vi "Finish.vi"   [LabVIEW 2019]
doc: "This VI is called just before exiting. It is expected to close I/O refnum, save collected data, etc."
uses:
  RefNums_Actuators.vi
  Joystick RefNum.vi
  RefNums_Sensors.vi
types:
  T1 = typedef "WPI_MotorControlDeviceRef.ctl" = cluster{"DeviceStatus":errorcluster, "Type":T2, "PWM":cluster{"PWM Channel":T3, "DeadBand":T4}, "CAN":cluster{"Device Number":u8, "SetOutput VI Ref":variant, "GetOutput VI Ref":variant, "Enable VI Ref":variant, "Disable VI Ref":variant, "Data":variant}, "Invert":bool, "DIO PWM":cluster{"PWM \"Enable\" Channel":T3, "DIOChannel":T5, "PWM Rate":dbl}}
  T2 = typedef "WPI_MotorControlType.ctl" = enum16{"PWM", "CAN", "DIO PWM"}
  T3 = typedef "FPGA_DIOPWMChannel.ctl" = enum8{"PWM 0", "PWM 1", "PWM 2", "PWM 3", "PWM 4", "PWM 5", "PWM 6", "PWM 7", "PWM 8", "PWM 9", "PWM MXP 0", "PWM MXP 1", "PWM MXP 2", "PWM MXP 3", "PWM MXP 4", "PWM MXP 5", "PWM MXP 6", "PWM MXP 7", "PWM MXP 8", "PWM MXP 9", "Invalid"}
  T4 = typedef "WPI_PWMDeadband.ctl" = cluster{"Name":string, "maxPositivePwm":i32, "minPositivePwm":i32, "centerPwm":i32, "maxNegativePwm":i32, "minNegativePwm":i32, "angularRange":u16}
  T5 = typedef "FPGA_DIOChannel.ctl" = enum8{"DIO 0", "DIO 1", "DIO 2", "DIO 3", "DIO 4", "DIO 5", "DIO 6", "DIO 7", "DIO 8", "DIO 9", "DIO MXP 0", "DIO MXP 1", "DIO MXP 2", "DIO MXP 3", "DIO MXP 4", "DIO MXP 5", "DIO MXP 6", "DIO MXP 7", "DIO MXP 8", "DIO MXP 9", "DIO MXP 10", "DIO MXP 11", "DIO MXP 12", "DIO MXP 13", "DIO MXP 14", "DIO MXP 15", "SPI Port CS1", "SPI Port CS2", "SPI Port CS3", "SPI Port MISO", "SPI Port MOSI", "Invalid"}
  T6 = typedef "WPI_JoystickDevRef.ctl" = cluster{"Device":T7}
  T7 = typedef "WPI_JoystickDeviceEnum.ctl" = enum16{"USB 0", "USB 1", "USB 2", "USB 3", "USB 4", "USB 5"}
  T8 = typedef "WPI_CompressorDevRef.ctl" = cluster{"DevStatus":errorcluster, "Pneumatics Control Module":u8}
  T9 = typedef "WPI_SolenoidDevRef.ctl" = cluster{"DevStatus":errorcluster, "Pneumatics Control Module":u8, "Forward Solenoid Channel":T10, "Reverse Solenoid Channel":T10}
  T10 = typedef "WPI_SolenoidChannel.ctl" = enum8{"Solenoid 0", "Solenoid 1", "Solenoid 2", "Solenoid 3", "Solenoid 4", "Solenoid 5", "Solenoid 6", "Solenoid 7", "Invalid"}
  T11 = typedef "WPI_AnalogChannelDevRef.ctl" = cluster{"DevStatus":errorcluster, "Analog Channel":T12}
  T12 = typedef "FPGA_AIChannel.ctl" = enum8{"AI 0", "AI 1", "AI 2", "AI 3", "AI MXP 0", "AI MXP 1", "AI MXP 2", "AI MXP 3", "Invalid"}
  T13 = typedef "WPI_ServoDeviceRef.ctl" = cluster{"DeviceStatus":errorcluster, "PWM Channel":T3, "DeadBand":T4}
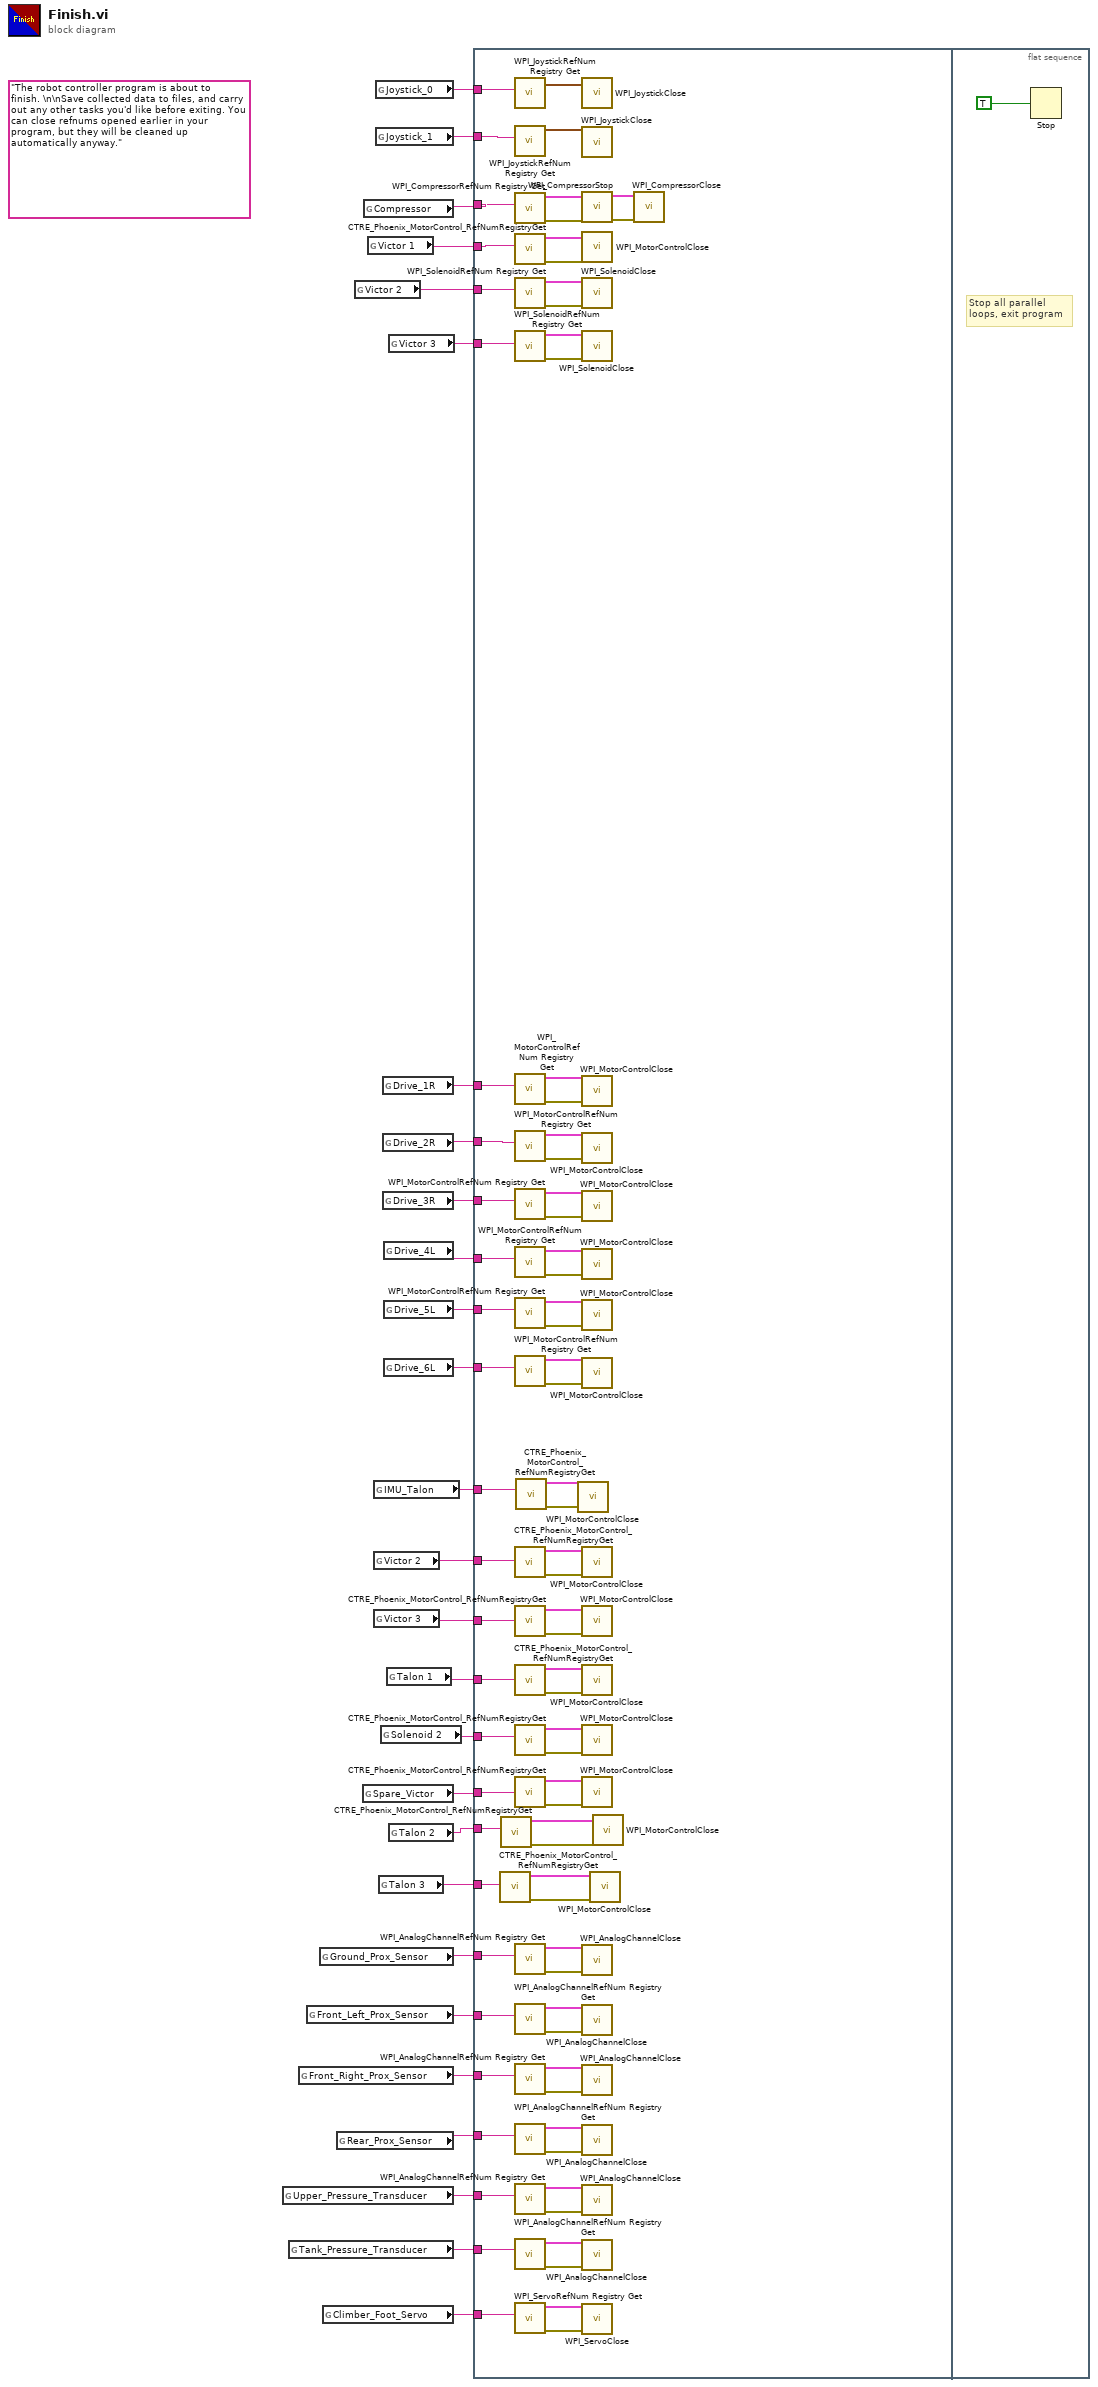
[diagram p0: block diagram]
diagram:
  (unwired) "The robot controller program is about to finish. \n\nSave collected data to files, and carry out any other tasks you'd like before exiting. You can close refnums opened earlier in your program, but they will be cleaned up automatically anyway."
  n1 = global read "RefNums_Sensors.vi" "Upper_Pressure_Transducer"() -> (w7:string)
  n2 = global read "RefNums_Sensors.vi" "Tank_Pressure_Transducer"() -> (w6:string)
  n3 = global read "RefNums_Sensors.vi" "Front_Right_Prox_Sensor"() -> (w9:string)
  n4 = global read "RefNums_Sensors.vi" "Front_Left_Prox_Sensor"() -> (w10:string)
  n5 = global read "RefNums_Sensors.vi" "Ground_Prox_Sensor"() -> (w24:string)
  n6 = global read "RefNums_Actuators.vi" "Climber_Foot_Servo"() -> (w23:string)
  n7 = global read "RefNums_Sensors.vi" "Rear_Prox_Sensor"() -> (w8:string)
  n8 = global read "RefNums_Actuators.vi" "Victor 2"() -> (w25:string)
  n9 = global read "RefNums_Actuators.vi" "Spare_Victor"() -> (w11:string)
  n10 = global read "RefNums_Actuators.vi" "Compressor"() -> (w27:string)
  n11 = global read "RefNums_Actuators.vi" "Victor 1"() -> (w26:string)
  n12 = global read "RefNums_Actuators.vi" "IMU_Talon"() -> (w3:string)
  n13 = global read "RefNums_Actuators.vi" "Victor 2"() -> (w15:string)
  n14 = global read "RefNums_Actuators.vi" "Victor 3"() -> (w14:string)
  n15 = global read "Joystick RefNum.vi" "Joystick_0"() -> (w5:string)
  n16 = global read "Joystick RefNum.vi" "Joystick_1"() -> (w4:string)
  n17 = global read "RefNums_Actuators.vi" "Talon 3"() -> (w1:string)
  n18 = global read "RefNums_Actuators.vi" "Solenoid 2"() -> (w12:string)
  n19 = global read "RefNums_Actuators.vi" "Drive_1R"() -> (w21:string)
  n20 = global read "RefNums_Actuators.vi" "Drive_2R"() -> (w20:string)
  n21 = global read "RefNums_Actuators.vi" "Drive_3R"() -> (w19:string)
  n22 = global read "RefNums_Actuators.vi" "Drive_4L"() -> (w18:string)
  n23 = global read "RefNums_Actuators.vi" "Drive_5L"() -> (w17:string)
  n24 = global read "RefNums_Actuators.vi" "Drive_6L"() -> (w16:string)
  n25 = global read "RefNums_Actuators.vi" "Talon 1"() -> (w13:string)
  n26 = global read "RefNums_Actuators.vi" "Victor 3"() -> (w22:string)
  n27 = global read "RefNums_Actuators.vi" "Talon 2"() -> (w2:string)
  n28 = flat-sequence {
    tunnel: w27 -> [w108]
    tunnel: w26 -> [w103]
    tunnel: w25 -> [w101]
    tunnel: w24 -> [w97]
    tunnel: w23 -> [w92]
    tunnel: w22 -> [w89]
    tunnel: w21 -> [w86]
    tunnel: w20 -> [w75]
    tunnel: w19 -> [w74]
    tunnel: w18 -> [w73]
    tunnel: w17 -> [w72]
    tunnel: w16 -> [w71]
    tunnel: w15 -> [w60]
    tunnel: w14 -> [w59]
    tunnel: w13 -> [w58]
    tunnel: w12 -> [w57]
    tunnel: w11 -> [w56]
    tunnel: w10 -> [w48]
    tunnel: w9 -> [w47]
    tunnel: w8 -> [w46]
    tunnel: w7 -> [w45]
    tunnel: w6 -> [w41]
    tunnel: w5 -> [w40]
    tunnel: w4 -> [w38]
    tunnel: w3 -> [w34]
    tunnel: w2 -> [w31]
    tunnel: w1 -> [w28]
    frame #0 {
      n29 = call <vilib>:"CTRE_Phoenix_MotorControl_RefNumRegistryGet.vi"("refnum name"=w28) -> ("error out"=w30:errorcluster, "PhoenixMotorControlDevRef"=w29:T1)  [unwired: 9 in]
      n30 = call <vilib>:"CTRE_Phoenix_MotorControl_RefNumRegistryGet.vi"("refnum name"=w31) -> ("error out"=w33:errorcluster, "PhoenixMotorControlDevRef"=w32:T1)  [unwired: 9 in]
      n31 = call <vilib>:"WPI_JoystickRefNum Registry Get.vi"("refnum name"=w40) -> ("JoystickDevRef"=w39:T6)  [unwired: 1 in, 9 out]
      n32 = call <vilib>:"WPI_JoystickRefNum Registry Get.vi"("refnum name"=w38) -> ("JoystickDevRef"=w37:T6)  [unwired: 1 in, 9 out]
      n33 = call <vilib>:"WPI_CompressorRefNum Registry Get.vi"("refnum name"=w108) -> ("error out"=w105:errorcluster, "CompressorDevRef"=w107:T8)  [unwired: 9 in]
      n34 = call <vilib>:"CTRE_Phoenix_MotorControl_RefNumRegistryGet.vi"("refnum name"=w103) -> ("error out"=w98:errorcluster, "PhoenixMotorControlDevRef"=w102:T1)  [unwired: 9 in]
      n35 = call <vilib>:"WPI_SolenoidRefNum Registry Get.vi"("refnum name"=w101) -> ("error out"=w99:errorcluster, "SolenoidDevRef"=w100:T9)  [unwired: 9 in]
      n36 = call <vilib>:"WPI_SolenoidRefNum Registry Get.vi"("refnum name"=w89) -> ("error out"=w91:errorcluster, "SolenoidDevRef"=w90:T9)  [unwired: 9 in]
      n37 = call <vilib>:"WPI_MotorControlRefNum Registry Get.vi"("refnum name"=w86) -> ("error out"=w87:errorcluster, "MotorControlDevRef"=w88:T1)  [unwired: 9 in]
      n38 = call <vilib>:"WPI_MotorControlRefNum Registry Get.vi"("refnum name"=w75) -> ("error out"=w85:errorcluster, "MotorControlDevRef"=w84:T1)  [unwired: 9 in]
      n39 = call <vilib>:"WPI_MotorControlRefNum Registry Get.vi"("refnum name"=w74) -> ("error out"=w83:errorcluster, "MotorControlDevRef"=w82:T1)  [unwired: 9 in]
      n40 = call <vilib>:"WPI_MotorControlRefNum Registry Get.vi"("refnum name"=w73) -> ("error out"=w81:errorcluster, "MotorControlDevRef"=w80:T1)  [unwired: 9 in]
      n41 = call <vilib>:"WPI_MotorControlRefNum Registry Get.vi"("refnum name"=w72) -> ("error out"=w76:errorcluster, "MotorControlDevRef"=w79:T1)  [unwired: 9 in]
      n42 = call <vilib>:"WPI_MotorControlRefNum Registry Get.vi"("refnum name"=w71) -> ("error out"=w78:errorcluster, "MotorControlDevRef"=w77:T1)  [unwired: 9 in]
      n43 = call <vilib>:"CTRE_Phoenix_MotorControl_RefNumRegistryGet.vi"("refnum name"=w60) -> ("error out"=w69:errorcluster, "PhoenixMotorControlDevRef"=w70:T1)  [unwired: 9 in]
      n44 = call <vilib>:"CTRE_Phoenix_MotorControl_RefNumRegistryGet.vi"("refnum name"=w59) -> ("error out"=w67:errorcluster, "PhoenixMotorControlDevRef"=w68:T1)  [unwired: 9 in]
      n45 = call <vilib>:"CTRE_Phoenix_MotorControl_RefNumRegistryGet.vi"("refnum name"=w58) -> ("error out"=w65:errorcluster, "PhoenixMotorControlDevRef"=w66:T1)  [unwired: 9 in]
      n46 = call <vilib>:"CTRE_Phoenix_MotorControl_RefNumRegistryGet.vi"("refnum name"=w57) -> ("error out"=w63:errorcluster, "PhoenixMotorControlDevRef"=w64:T1)  [unwired: 9 in]
      n47 = call <vilib>:"CTRE_Phoenix_MotorControl_RefNumRegistryGet.vi"("refnum name"=w56) -> ("error out"=w61:errorcluster, "PhoenixMotorControlDevRef"=w62:T1)  [unwired: 9 in]
      n48 = call <vilib>:"WPI_AnalogChannelRefNum Registry Get.vi"("refnum name"=w97) -> ("error out"=w95:errorcluster, "AIDeviceRef"=w96:T11)  [unwired: 9 in]
      n49 = call <vilib>:"WPI_AnalogChannelRefNum Registry Get.vi"("refnum name"=w48) -> ("error out"=w55:errorcluster, "AIDeviceRef"=w54:T11)  [unwired: 9 in]
      n50 = call <vilib>:"WPI_AnalogChannelRefNum Registry Get.vi"("refnum name"=w47) -> ("error out"=w53:errorcluster, "AIDeviceRef"=w52:T11)  [unwired: 9 in]
      n51 = call <vilib>:"WPI_AnalogChannelRefNum Registry Get.vi"("refnum name"=w46) -> ("error out"=w50:errorcluster, "AIDeviceRef"=w49:T11)  [unwired: 9 in]
      n52 = call <vilib>:"WPI_AnalogChannelRefNum Registry Get.vi"("refnum name"=w45) -> ("error out"=w44:errorcluster, "AIDeviceRef"=w51:T11)  [unwired: 9 in]
      n53 = call <vilib>:"WPI_AnalogChannelRefNum Registry Get.vi"("refnum name"=w41) -> ("error out"=w43:errorcluster, "AIDeviceRef"=w42:T11)  [unwired: 9 in]
      n54 = call <vilib>:"WPI_ServoRefNum Registry Get.vi"("refnum name"=w92) -> ("error out"=w94:errorcluster, "ServoDeviceRef"=w93:T13)  [unwired: 9 in]
      n55 = call <vilib>:"CTRE_Phoenix_MotorControl_RefNumRegistryGet.vi"("refnum name"=w34) -> ("error out"=w35:errorcluster, "PhoenixMotorControlDevRef"=w36:T1)  [unwired: 9 in]
      n56 = call <vilib>:"WPI_MotorControlClose.vi"("error in"=w35, "MotorControlDevRef"=w36) -> ()  [unwired: 9 in, 1 out]
      n57 = call <vilib>:"WPI_JoystickClose.vi"("JoystickDevRef"=w39) -> ()  [unwired: 11 out]
      n58 = call <vilib>:"WPI_JoystickClose.vi"("JoystickDevRef"=w37) -> ()  [unwired: 11 out]
      n59 = call <vilib>:"WPI_CompressorStop.vi"("error in (no error)"=w105, "CompressorDevRef"=w107) -> ("error out"=w104:errorcluster, "CompressorDevRef"=w106:T8)  [unwired: 8 in]
      n60 = call <vilib>:"WPI_MotorControlClose.vi"("error in"=w98, "MotorControlDevRef"=w102) -> ()  [unwired: 9 in, 1 out]
      n61 = call <vilib>:"WPI_SolenoidClose.vi"("error in (no error)"=w99, "SolenoidDevRef"=w100) -> ()  [unwired: 9 in, 1 out]
      n62 = call <vilib>:"WPI_SolenoidClose.vi"("error in (no error)"=w91, "SolenoidDevRef"=w90) -> ()  [unwired: 9 in, 1 out]
      n63 = call <vilib>:"WPI_MotorControlClose.vi"("error in"=w87, "MotorControlDevRef"=w88) -> ()  [unwired: 9 in, 1 out]
      n64 = call <vilib>:"WPI_MotorControlClose.vi"("error in"=w85, "MotorControlDevRef"=w84) -> ()  [unwired: 9 in, 1 out]
      n65 = call <vilib>:"WPI_MotorControlClose.vi"("error in"=w83, "MotorControlDevRef"=w82) -> ()  [unwired: 9 in, 1 out]
      n66 = call <vilib>:"WPI_MotorControlClose.vi"("error in"=w81, "MotorControlDevRef"=w80) -> ()  [unwired: 9 in, 1 out]
      n67 = call <vilib>:"WPI_MotorControlClose.vi"("error in"=w76, "MotorControlDevRef"=w79) -> ()  [unwired: 9 in, 1 out]
      n68 = call <vilib>:"WPI_MotorControlClose.vi"("error in"=w78, "MotorControlDevRef"=w77) -> ()  [unwired: 9 in, 1 out]
      n69 = call <vilib>:"WPI_MotorControlClose.vi"("error in"=w69, "MotorControlDevRef"=w70) -> ()  [unwired: 9 in, 1 out]
      n70 = call <vilib>:"WPI_MotorControlClose.vi"("error in"=w67, "MotorControlDevRef"=w68) -> ()  [unwired: 9 in, 1 out]
      n71 = call <vilib>:"WPI_MotorControlClose.vi"("error in"=w65, "MotorControlDevRef"=w66) -> ()  [unwired: 9 in, 1 out]
      n72 = call <vilib>:"WPI_MotorControlClose.vi"("error in"=w63, "MotorControlDevRef"=w64) -> ()  [unwired: 9 in, 1 out]
      n73 = call <vilib>:"WPI_MotorControlClose.vi"("error in"=w61, "MotorControlDevRef"=w62) -> ()  [unwired: 9 in, 1 out]
      n74 = call <vilib>:"WPI_AnalogChannelClose.vi"("error in (no error)"=w95, "AIDeviceRef"=w96) -> ()  [unwired: 9 in, 1 out]
      n75 = call <vilib>:"WPI_AnalogChannelClose.vi"("error in (no error)"=w55, "AIDeviceRef"=w54) -> ()  [unwired: 9 in, 1 out]
      n76 = call <vilib>:"WPI_AnalogChannelClose.vi"("error in (no error)"=w53, "AIDeviceRef"=w52) -> ()  [unwired: 9 in, 1 out]
      n77 = call <vilib>:"WPI_AnalogChannelClose.vi"("error in (no error)"=w50, "AIDeviceRef"=w49) -> ()  [unwired: 9 in, 1 out]
      n78 = call <vilib>:"WPI_AnalogChannelClose.vi"("error in (no error)"=w44, "AIDeviceRef"=w51) -> ()  [unwired: 9 in, 1 out]
      n79 = call <vilib>:"WPI_AnalogChannelClose.vi"("error in (no error)"=w43, "AIDeviceRef"=w42) -> ()  [unwired: 9 in, 1 out]
      n80 = call <vilib>:"WPI_ServoClose.vi"("error in (no error)"=w94, "ServoDeviceRef"=w93) -> ()  [unwired: 9 in, 1 out]
      n81 = call <vilib>:"WPI_MotorControlClose.vi"("error in"=w30, "MotorControlDevRef"=w29) -> ()  [unwired: 9 in, 1 out]
      n82 = call <vilib>:"WPI_MotorControlClose.vi"("error in"=w33, "MotorControlDevRef"=w32) -> ()  [unwired: 9 in, 1 out]
      n83 = call <vilib>:"WPI_CompressorClose.vi"("error in (no error)"=w104, "CompressorDevRef"=w106) -> ()  [unwired: 9 in, 1 out]
    }
    frame #1 {
      # "Stop all parallel\nloops, exit program"
      n84 = Stop(stop? (T)=TRUE ("Quit")) -> ()
    }
  }
